vi "Process.vi"(8 "error in":errorcluster, 11 "Example Instrument UI":refnum<class "Instrument.PPMS UI.lvclass">) -> (0 "error out":errorcluster, 3 "Example Instrument UI out":refnum<class "Instrument.PPMS UI.lvclass">)   [LabVIEW 2016, in "Instrument.PPMS UI.lvclass"]
doc: "---------------------------------------------------------------\nJKI State Machine Objects™\nhttp://jki.net/state-machine-objects/\nCopyright (C) 2005-2015, JKI <info@jki.net>\nALL RIGHTS RESERVEDJKI State Machine Objects (SMO) 1.0.0.5\nJKI - JKI\nCopyright (c) 2016, JKI"
uses:
  Instrument.PPMS UI.lvclass
  C:/Program Files (x86)/National Instruments/LabVIEW 2016/vi.lib/JKI/JKI SMO/SMO/SMO.lvclass
  C:/Program Files (x86)/National Instruments/LabVIEW 2016/vi.lib/JKI/JKI SMO/SMO.UI/SMO.UI.lvclass
  instrument.PPMS/Typedefs/Magnet Status--PPMS--ring.ctl
  instrument.PPMS/Typedefs/Temperature Status--PPMS--ring.ctl
  <vilib>/JKI/JKI SMO/SMO/Typedefs/Parent Call--Enum.ctl
  instrument.PPMS/instrument.PPMS.lvclass
  C:/Program Files (x86)/National Instruments/LabVIEW 2016/user.lib/LevyLab/Levylab Instruments/SMOs/Instrument/Instrument.lvclass
  Instrument.PPMS UI.lvclass/Instrument.PPMS UI.ctl
  instrument.PPMS/Typedefs/getAll--PPMS--cluster.ctl
  <vilib>/JKI/JKI SMO/SMO.UI/SMO.UI.lvclass
  <vilib>/JKI/JKI SMO/SMO/SMO.lvclass
  <userlib>/LevyLab/Levylab Instruments/SMOs/Instrument/Instrument.lvclass
panel:
  in  "Field":bool
  in  "Temperature":bool
  in  "Target Field (Oe)":dbl=-0.00643419474363327 format="%_3g"
  in  "Target Temperature (K)":dbl=305.0156 format="%#_5g"
  out "PPMS 1 Temperature Status":T1 items=["TemperatureUnknown"=0, "Stable"=1, "Tracking"=2, "Near"=5, "Chasing"=6, "Filling"=7, "Standby"=10, "Disabled"=13, "ImpedanceNotFunction"=14, "TempFailure"=15]
  out "PPMS 1 Magnet Status":T2=1 items=["MagnetUnknown"=0, "StablePersistent"=1, "WarmingSwitch"=2, "CoolingSwitch"=3, "StableDriven"=4, "Iterating"=5, "Charging"=6, "Discharging"=7, "CurrentError"=8, "MagnetFailure"=15]
  out "Helium Level (%)":dbl=86.7
  out "Field (Oe)":dbl=-0.00643419474363327 format="%_3g"
  out "Temperature(K)":dbl=305.0156 format="%#_5g"
  in  "update time (ms)":u32=200
  in  "STOP":bool
  # "PPMS Monitor"
  # "SMO UI Template"
  # "For instructions on how to use the JKI State Machine Objects, examples and video tutorials, visit:\nhttp://jki.net/state-machine-objects/\n\nJKI State Machine Objects™\nhttp://jki.net/state-machine-objects/\nCopyright (C) 2005-2015, JKI <info@jki.net>\nALL RIGHTS RESERVED"
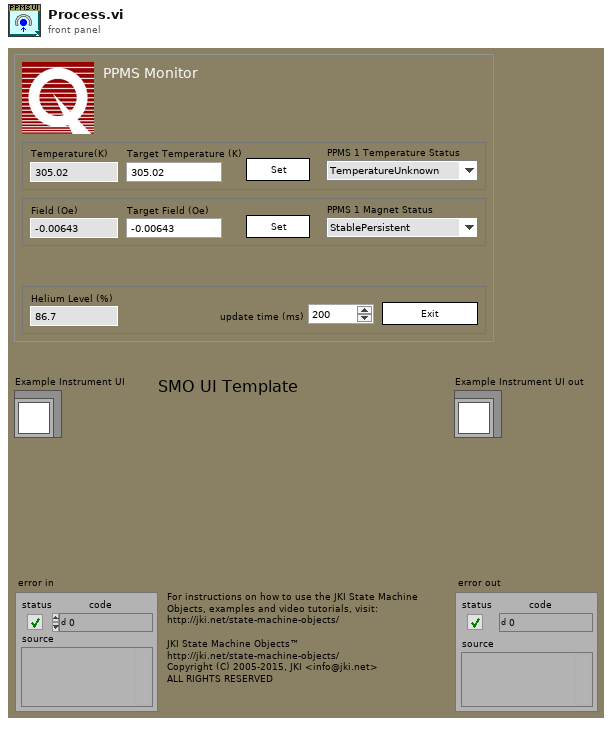
[diagram p1: front panel]
types:
  T1 = typedef "instrument.PPMS.lvclass/Temperature Status--PPMS--ring.ctl" = i32
  T2 = typedef "instrument.PPMS.lvclass/Magnet Status--PPMS--ring.ctl" = i32
  T3 = typedef "SMO.lvclass/Parent Call--Enum.ctl" = enum16{"Allows parent to run", "Does not request parent to run"}
  T4 = enum32{"invalid app kind", "Development System", "Run Time System", "Student Edition", "Embedded LabVIEW", "Evaluation", "Custom"}
  T5 = enum32{"Invalid", "Standard", "Closed", "Hidden", "Minimized", "Maximized"}
  T6 = typedef "instrument.PPMS.lvclass/getAll--PPMS--cluster.ctl" = cluster{"PPMS 1 Helium Level":dbl, "PPMS 1 Temperature":dbl, "PPMS 1 Temperature Status":T1, "PPMS 1 Magnetic Field":dbl, "PPMS 1 Magnet Status":T2}
  T7 = cluster{"Core":cluster{"Current VI Reference":refnum<vi>, "Close Panel on Exit?":bool, "error":errorcluster}, "Self Reference":refnum<class "Instrument.PPMS UI.lvclass">, "instrument.PPMS":refnum<class "instrument.PPMS.lvclass">, "Data Send":variant, "Data Receive":variant}
  T8 = cluster{"Current VI Reference":refnum<vi>, "Close Panel on Exit?":bool, "error":errorcluster}
  T9 = typedef "SMO.lvclass/Protected Events.ctl" = cluster{"StopProcesses":refnum<user-event>, "AbortProcesses":refnum<user-event>, "Config Changed":refnum<user-event>, "Dependency":refnum<user-event>}
  T10 = typedef "Instrument.lvclass/PublicEvents--Cluster.ctl" = cluster{"MessageFromProcess":refnum<user-event>}
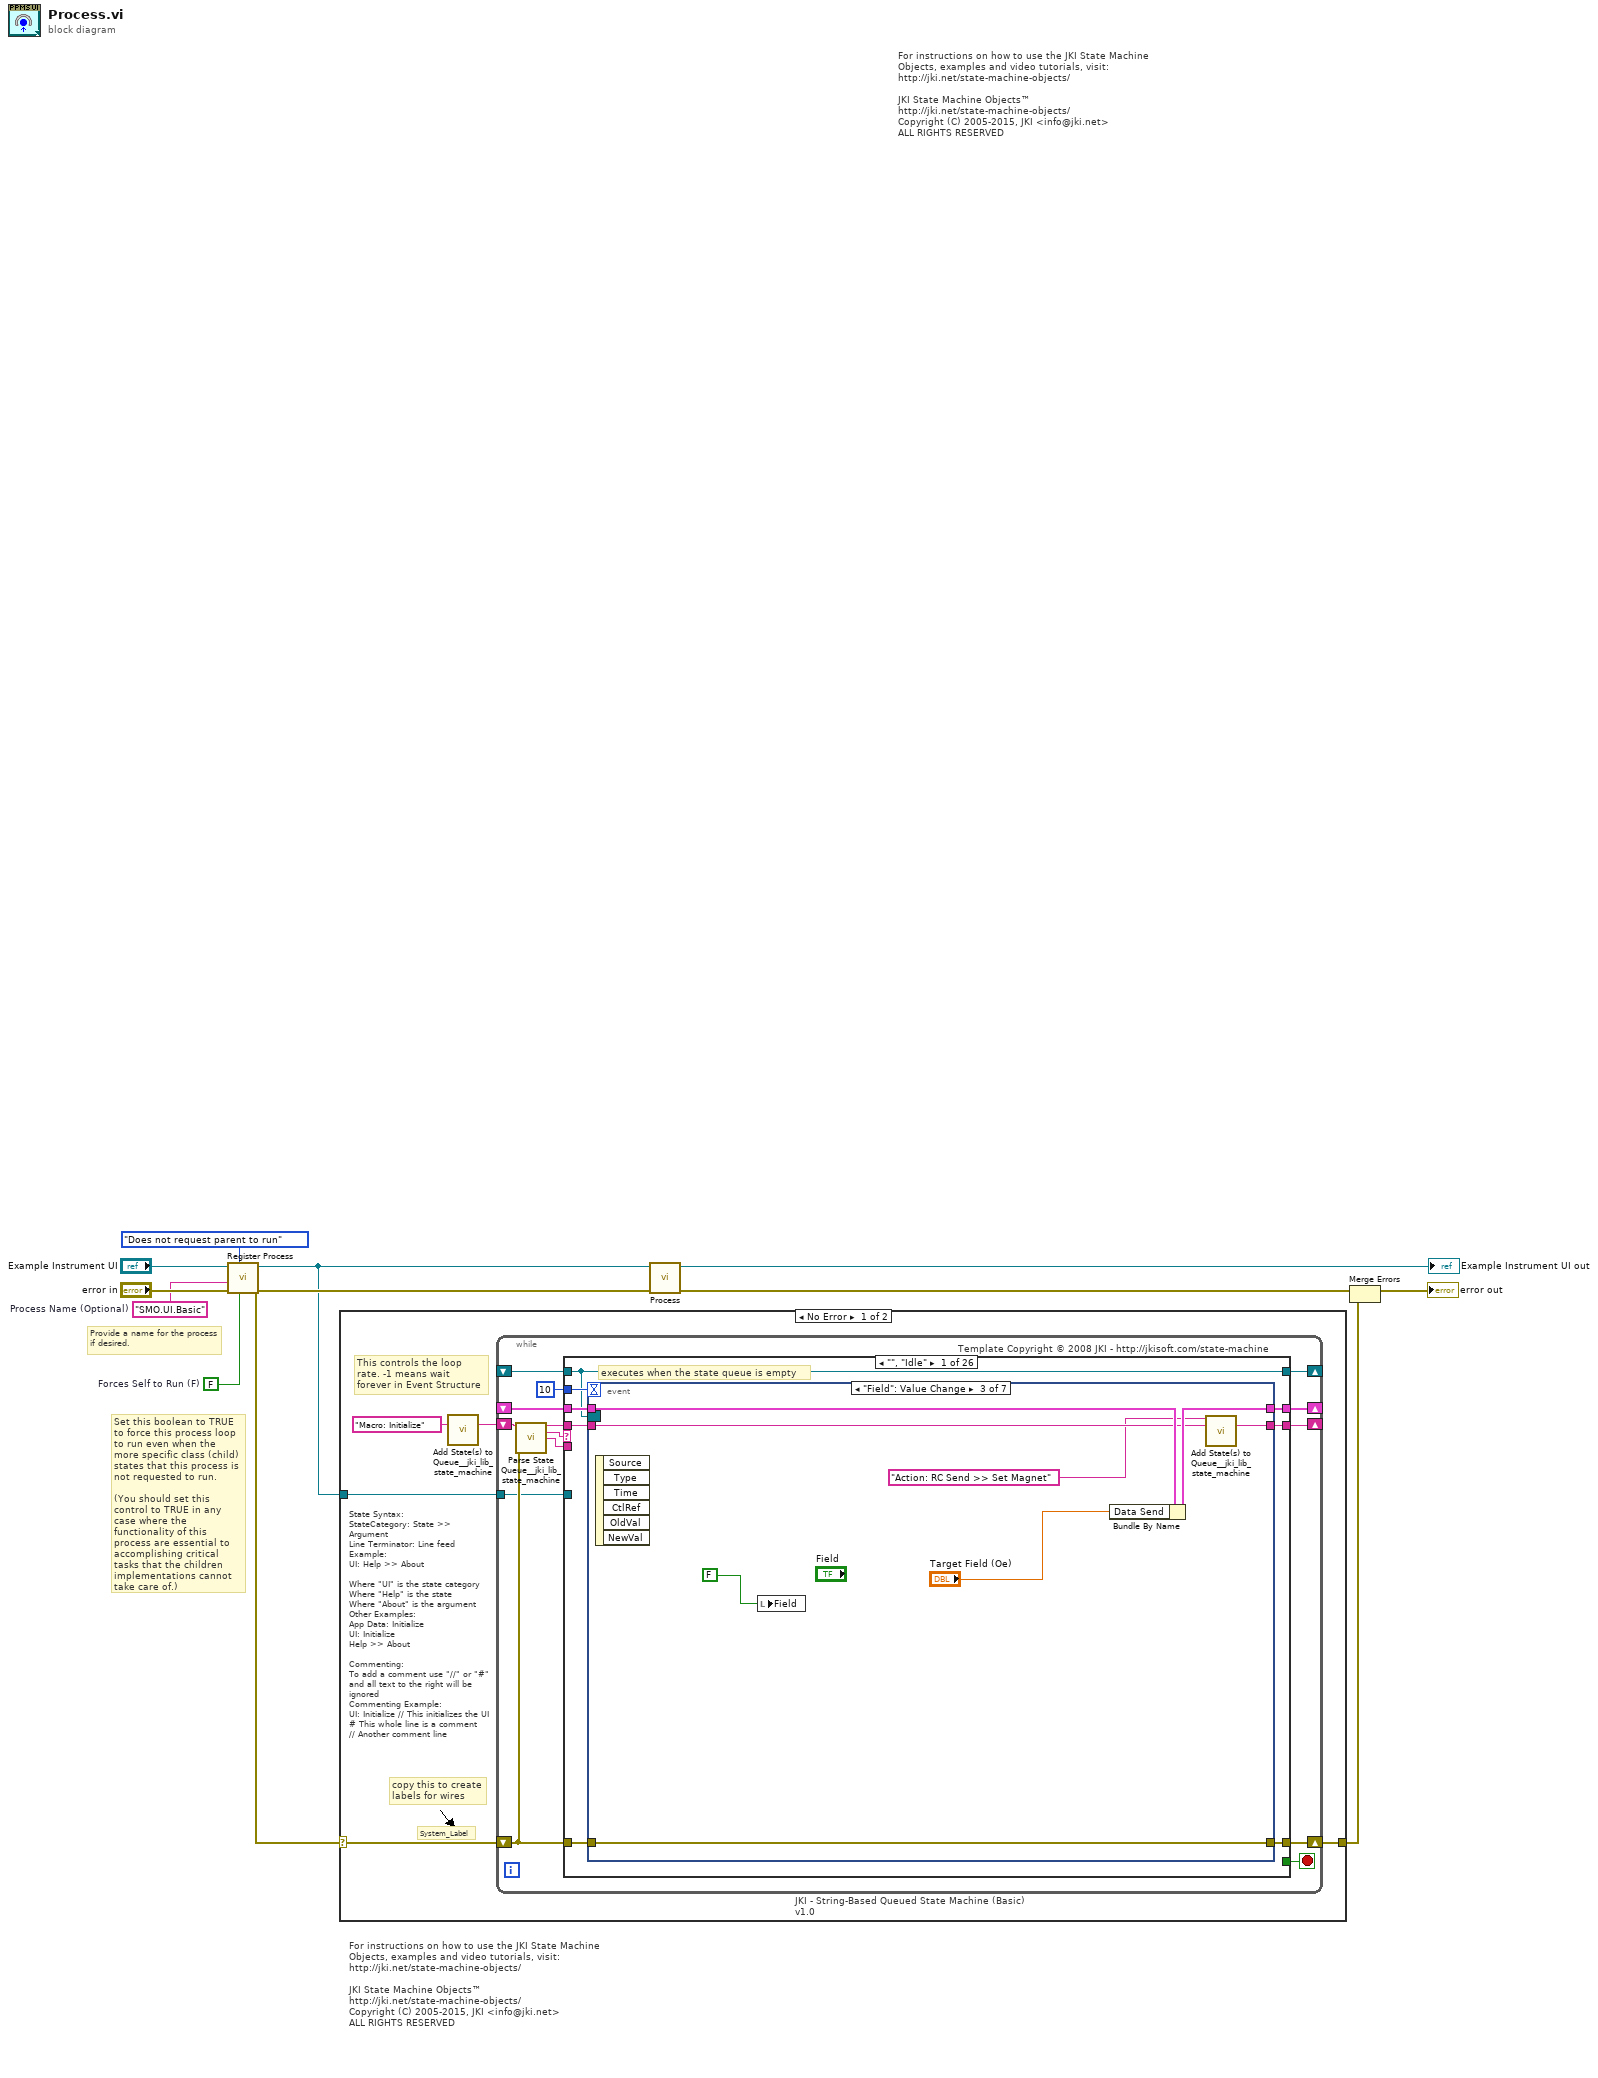
[diagram p0: block diagram]
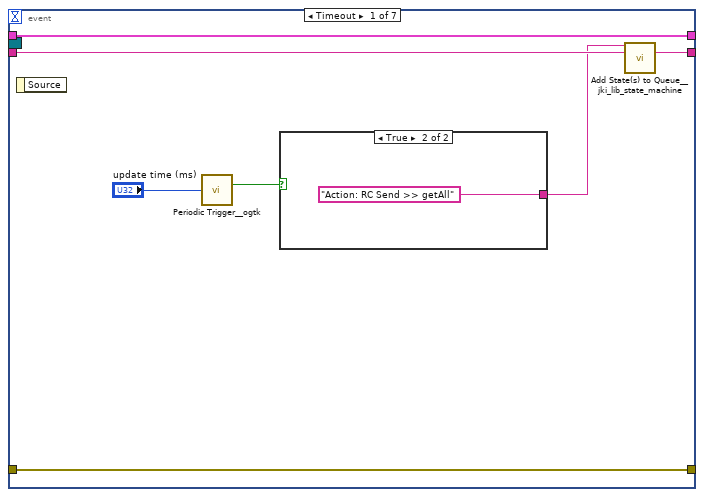
[diagram p2: hidden frame]
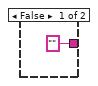
[diagram p3: hidden frame]
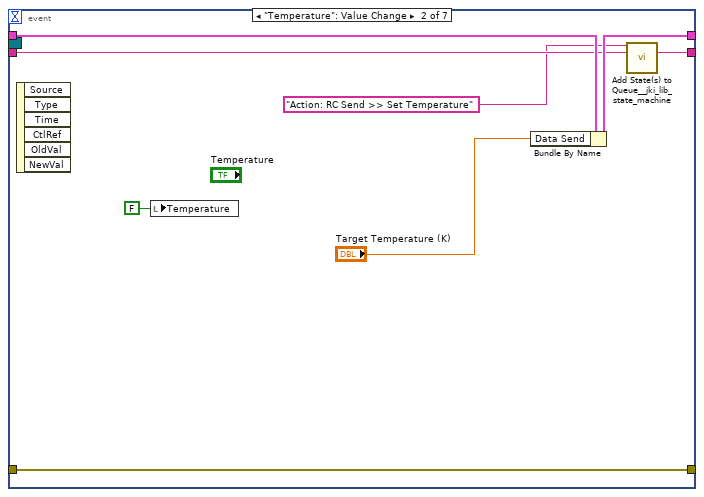
[diagram p4: hidden frame]
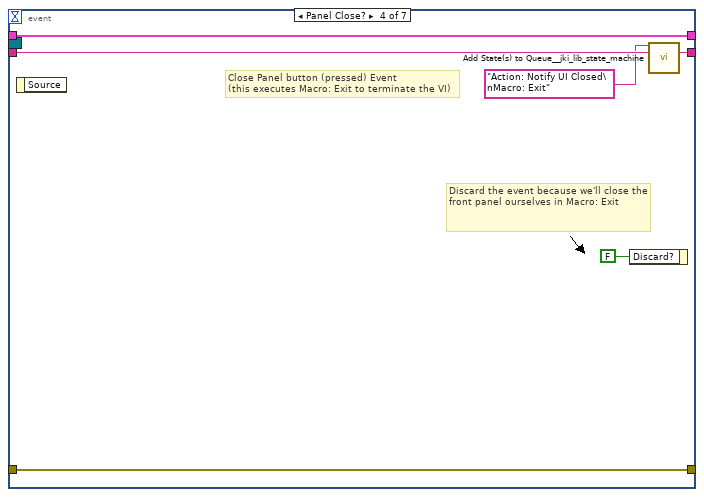
[diagram p5: hidden frame]
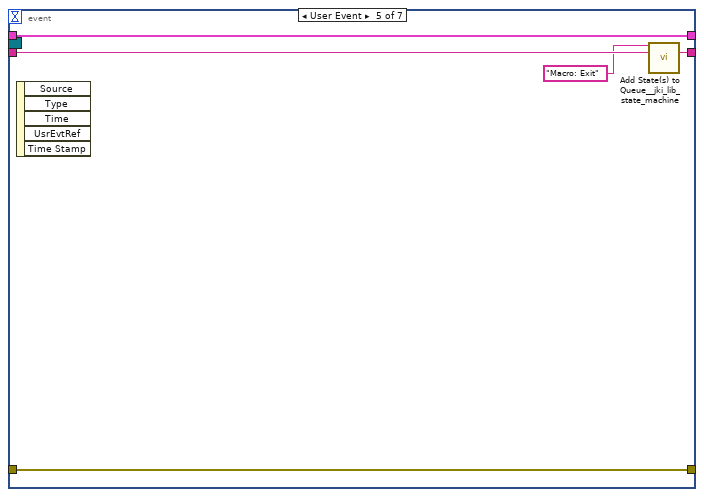
[diagram p6: hidden frame]
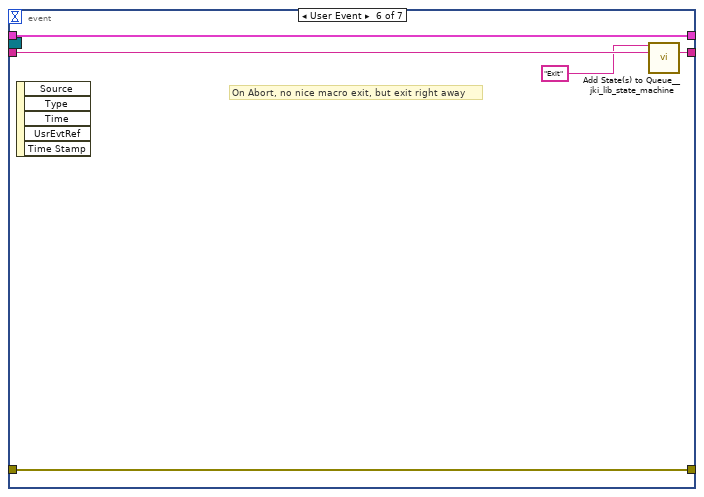
[diagram p7: hidden frame]
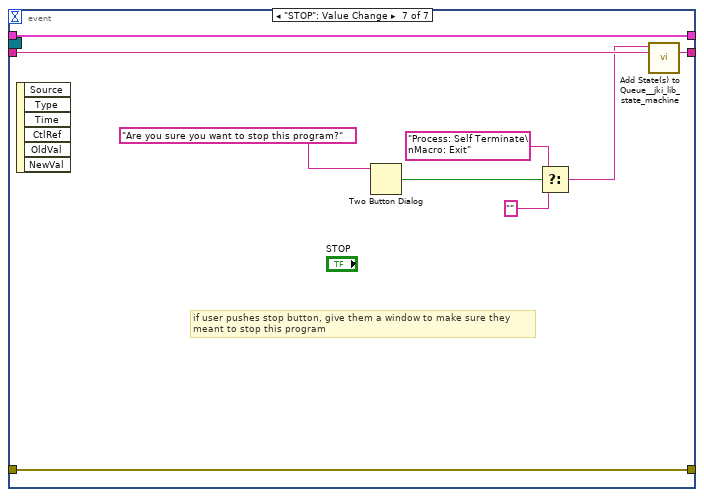
[diagram p8: hidden frame]
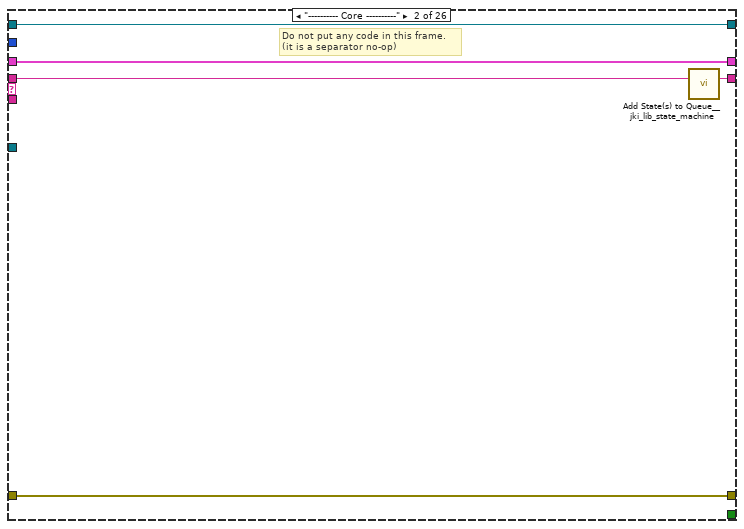
[diagram p9: hidden frame]
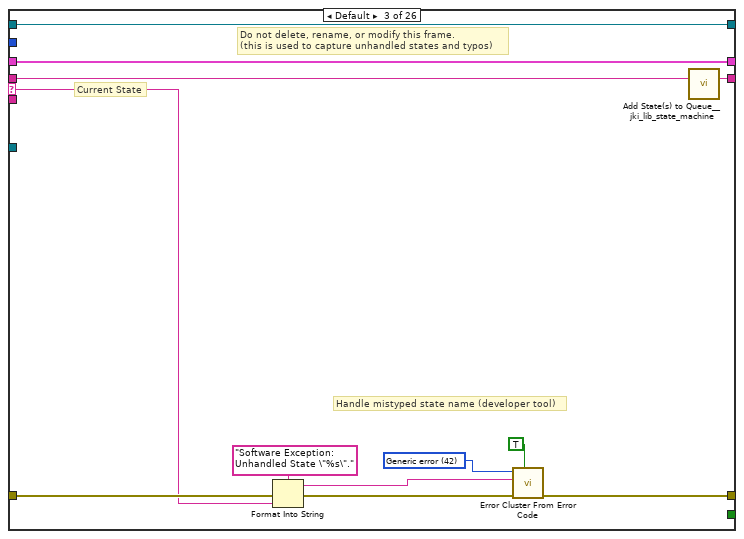
[diagram p10: hidden frame]
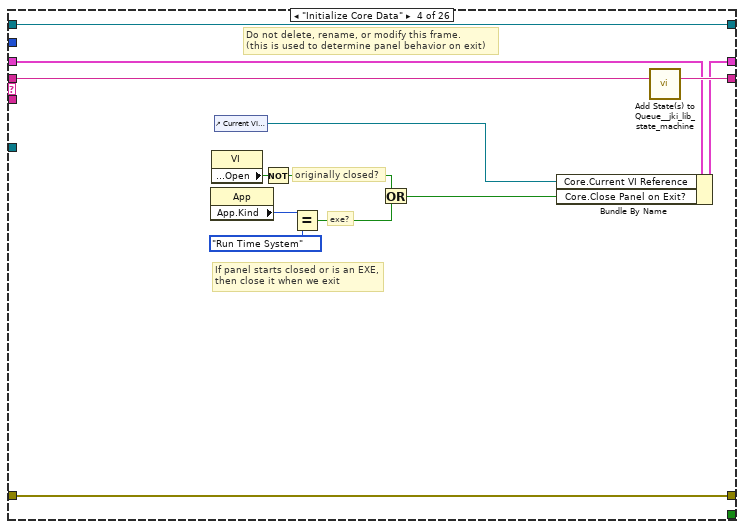
[diagram p11: hidden frame]
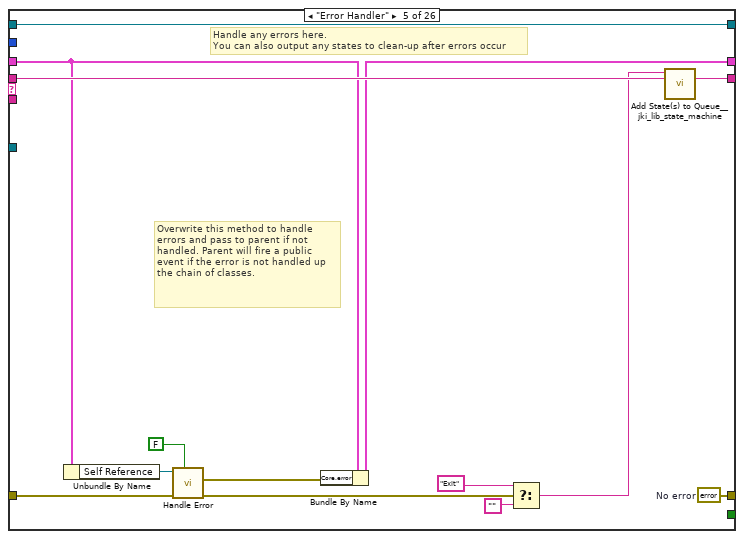
[diagram p12: hidden frame]
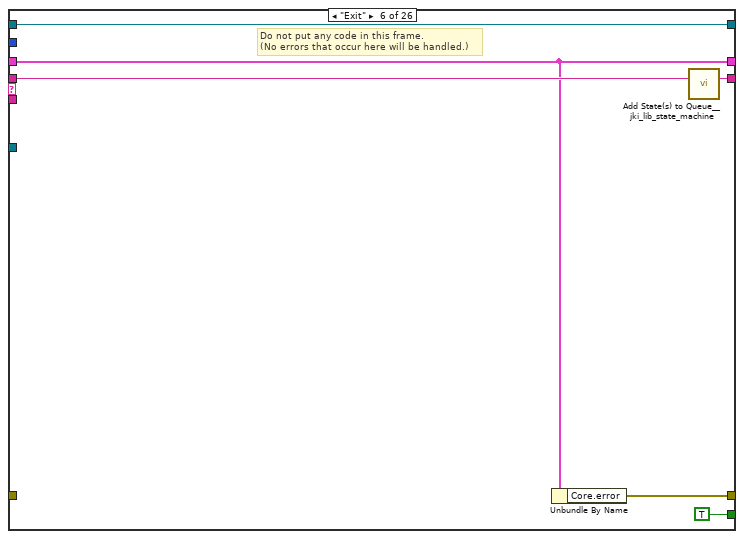
[diagram p13: hidden frame]
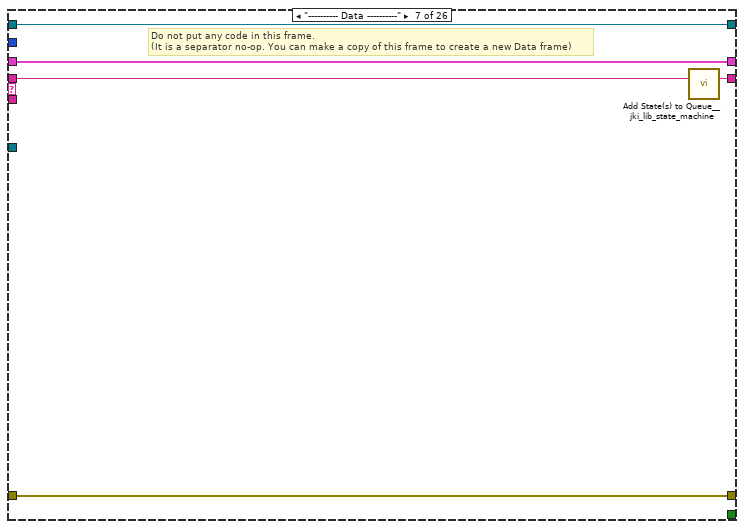
[diagram p14: hidden frame]
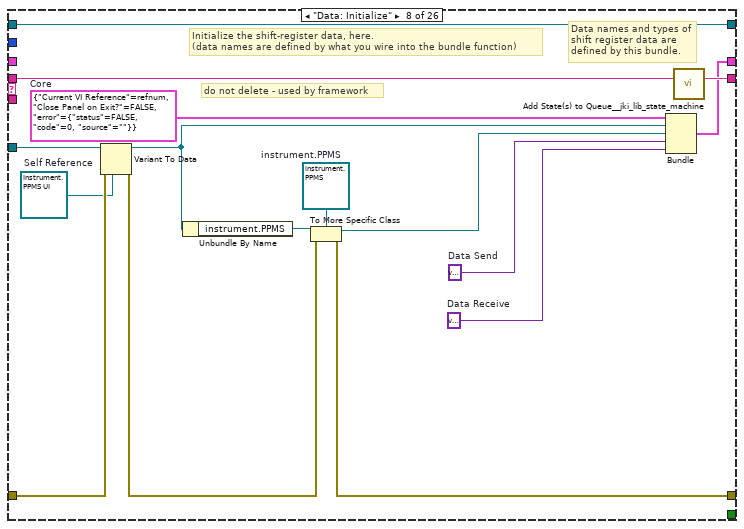
[diagram p15: hidden frame]
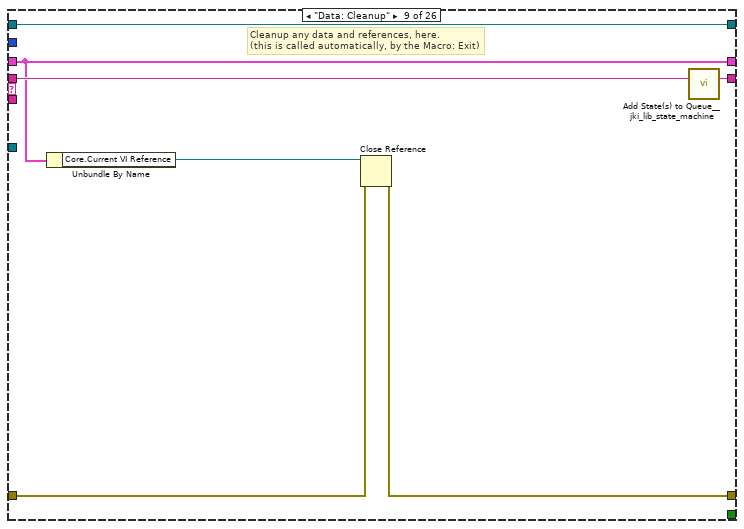
[diagram p16: hidden frame]
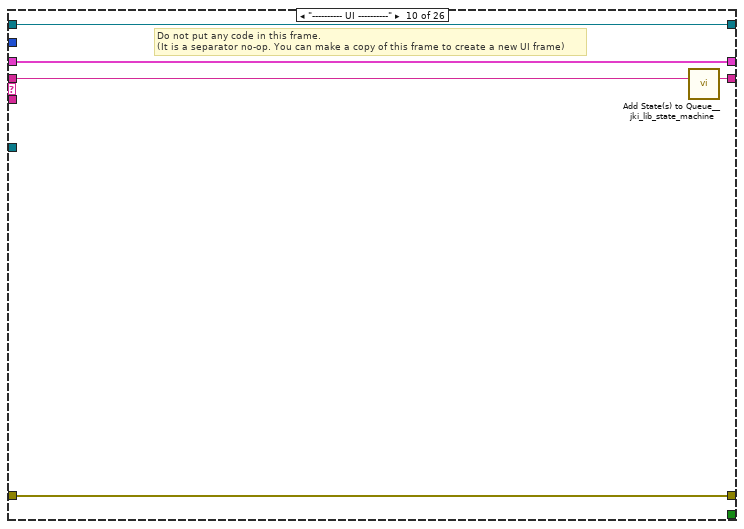
[diagram p17: hidden frame]
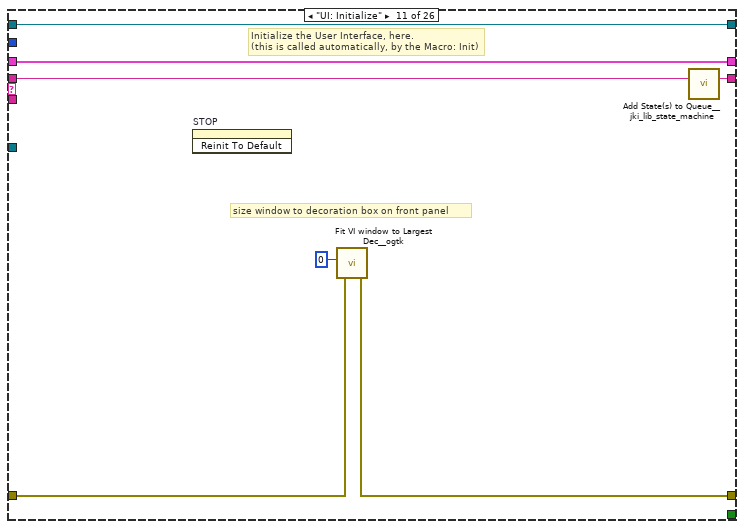
[diagram p18: hidden frame]
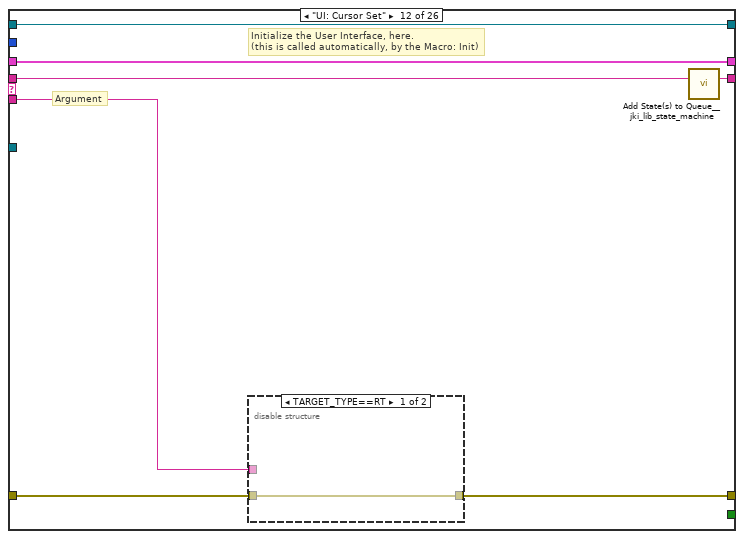
[diagram p19: hidden frame]
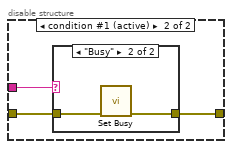
[diagram p20: hidden frame]
diagram:
  w2 = FALSE  # Forces Self to Run (F)
  w1 = "SMO.UI.Basic"  # Process Name (Optional)
  # "For instructions on how to use the JKI State Machine Objects, examples and video tutorials, visit:\nhttp://jki.net/state-machine-objects/\n\nJKI State Machine Objects™\nhttp://jki.net/state-machine-objects/\nCopyright (C) 2005-2015, JKI <info@jki.net>\nALL RIGHTS RESERVED"
  # "Provide a name for the process\nif desired."
  # "Set this boolean to TRUE to force this process loop to run even when the more specific class (child) states that this process is not requested to run.\n\n(You should set this control to TRUE in any case where the functionality of this process are essential to accomplishing critical tasks that the children implementations cannot take care of.)"
  # "For instructions on how to use the JKI State Machine Objects, examples and video tutorials, visit:\nhttp://jki.net/state-machine-objects/\n\nJKI State Machine Objects™\nhttp://jki.net/state-machine-objects/\nCopyright (C) 2005-2015, JKI <info@jki.net>\nALL RIGHTS RESERVED"
  n1 = call <vilib>:"Register Process.vi"("Forces Self to Run (F)"=w2, "Parent Call"=Parent_Call--Enum."Does not request parent to run", "error in (no error)"="error in", "Process Name (optional)"=w1, "SMO"="Example Instrument UI") -> ("error out"=w8:errorcluster, "SMO out"=w7:refnum<class "Instrument.PPMS UI.lvclass">)  [unwired: 5 in]
  n2 = case shown="No Error" w8 {
    selector: w8 -> [w13 w350]
    tunnel: w7 -> [w14 _]
    tunnel: [w12 w350] -> w4
    frame No Error {
      # "State Syntax:\nStateCategory: State >> Argument\nLine Terminator: Line feed\nExample:\nUI: Help >> About\n\nWhere \"UI\" is the state category\nWhere \"Help\" is the state\nWhere \"About\" is the argument\nOther Examples:\nApp Data: Initialize\nUI: Initialize\nHelp >> About\n\nCommenting:\nTo add a comment use \"//\" or \"#\" and all text to the right will be ignored\nCommenting Example:\nUI: Initialize // This initializes the UI\n# This whole line is a comment\n// Another comment line"
      # "copy this to create labels for wires"
      # "This controls the loop rate. -1 means wait forever in Event Structure"
      # "System_Label"
      n3 = call <vilib>:"Add State(s) to Queue__jki_lib_state_machine.vi"("State(s) in (\"\")"="Macro: Initialize") -> ("States Out"=w16:string)  [unwired: 14 in]
      n4 = while "JKI - String-Based Queued State Machine (Basic) v1.0" {
        shift-right: [w23] -> _
        shift-left: _ -> [w22]
        shift-right: [w26] -> w12
        shift-left: w13 -> [w20]
        shift-right: [w25] -> _
        shift-left: w16 -> [w27]
        tunnel: w14 -> [w19]
        shift-right: [w18] -> _
        shift-left: _ -> [w17]
        stop <- w24 stop-if-true
        # "Template Copyright © 2008 JKI - http://jkisoft.com/state-machine"
        n5 = call <vilib>:"Parse State Queue__jki_lib_state_machine.vi"("State Queue"=w27, "Error In (no error)"=w20) -> ("Remaining States"=w29:string, "Current State"=w30:string, "Arguments"=w28:string)  [unwired: 11 in]
        n6 = case shown="\"\", \"Idle\"" w30 {
          selector: w30 -> [_ _ w95 _ _ _ _ _ _ _ _ _ _ _ _ _ _ _ _ _ _ _ _ _ _ _]
          tunnel: w29 -> [w38 w93 w99 w118 w132 w138 w143 w159 w166 w171 w178 w185 w201 w233 w242 w256 w261 w272 w279 w284 w297 w303 w310 w317 w331 w345]
          tunnel: w28 -> [_ _ _ _ _ _ _ _ _ _ _ w179 w195 _ _ _ _ _ _ _ _ _ _ _ _ w336]
          tunnel: w22 -> [w36 w90 w97 w109 w120 w134 w140 _ w162 w168 w176 w183 w197 w230 w238 w247 w258 w269 w274 w281 w295 w301 w306 w313 w328 w342]
          tunnel: [w35 w91 w101 w115 w125 w133 w141 w145 w163 w169 w173 w180 w198 w231 w240 w254 w259 w263 w275 w282 w290 w298 w307 w311 w326 w334] -> w26
          tunnel: w20 -> [w34 w91 w100 w115 w121 _ w141 w156 w160 w169 w174 w181 w199 w231 w240 w254 w259 w264 w276 w282 w292 w299 w307 w312 w327 w335]
          tunnel: [w37 w92 w98 w117 w131 w137 w142 w158 w165 w170 w177 w184 w200 w232 w241 w255 w260 w271 w278 w283 w296 w302 w309 w316 w330 w344] -> w25
          tunnel: [_ _ _ _ _ TRUE _ _ _ _ _ _ _ _ _ _ _ _ _ _ _ _ _ _ _ _] -> w24
          tunnel: [w33 w90 w97 w116 w123 w134 w140 w157 w162 w168 w176 w183 w197 w230 w238 w247 w258 w269 w274 w281 w295 w301 w305 w313 w328 w341] -> w23
          tunnel: 10 ("Timeout") -> [w32 _ _ _ _ _ _ _ _ _ _ _ _ _ _ _ _ _ _ _ _ _ _ _ _ _]
          tunnel: w19 -> [_ _ _ _ _ _ _ w154 _ _ _ _ _ _ _ _ _ _ _ _ _ _ _ _ _ _]
          tunnel: [w31 w89 w94 w106 w130 w135 w139 w153 w161 w167 w175 w182 w194 w229 w239 w248 w257 w270 w277 w280 w294 w300 w308 w315 w329 w343] -> w18
          tunnel: w17 -> [w31 w89 w94 w106 w130 w135 w139 w153 w161 w167 w175 w182 w194 w229 w239 w248 w257 w270 w277 w280 _ w300 w308 w315 w329 w343]
          frame "", "Idle" {
            # "executes when the state queue is empty"
            n7 = event shown="[2] \"Field\": Value Change" {
              selector: w31 -> [_ _ _ _ _ _ _]
              dyn-events: _ -> [_ _ _ _ _ _ _]
              timeout: w32 -> [_ _ _ _ _ _ _]
              tunnel: w38 -> [w45 w51 w59 w69 w74 w79 w88]
              tunnel: [w44 w54 w62 w68 w73 w78 w87] -> w37
              tunnel: w36 -> [w42 w53 w61 w65 w71 w76 w85]
              tunnel: [w43 w55 w63 w64 w72 w77 w86] -> w35
              tunnel: w34 -> [w43 w55 w63 w64 w72 w77 w86]
              tunnel: [w42 w52 w60 w65 w71 w76 w85] -> w33
              event Timeout {
                n8 = event-data() -> ()  [unwired: 1 in, 1 out]
                n9 = call <userlib>:"Periodic Trigger__ogtk.vi"("time (ms)"="update time (ms)") -> ("Triggered"=w41:bool)  [unwired: 12 in, 2 out]
                n10 = case shown="True" w41 {
                  tunnel: ["" "Action: RC Send >> getAll"] -> w39
                  frame False {
                  }
                  frame True {
                  }
                }
                n11 = call <vilib>:"Add State(s) to Queue__jki_lib_state_machine.vi"("State(s) in Front (\"\")"=w39, "State(s) in (\"\")"=w45) -> ("States Out"=w44:string)  [unwired: 13 in]
              }
              event "Temperature": Value Change {
                n12 = event-data() -> ()  [unwired: 1 in, 6 out]
                n13 = local write "Temperature"(FALSE ("Temperature")) -> ()
                n14 = Bundle By Name(cluster=w53, "Data Send"="Target Temperature (K)") -> (w52:T7)
                n15 = call <vilib>:"Add State(s) to Queue__jki_lib_state_machine.vi"("State(s) in Front (\"\")"="Action: RC Send >> Set Temperature" ("State(s) in Front (\"\")"), "State(s) in (\"\")"=w51) -> ("States Out"=w54:string)  [unwired: 13 in]
              }
              event "Field": Value Change {
                n16 = event-data() -> ()  [unwired: 1 in, 6 out]
                n17 = local write "Field"(FALSE ("Field")) -> ()
                n18 = Bundle By Name(cluster=w61, "Data Send"="Target Field (Oe)") -> (w60:T7)
                n19 = call <vilib>:"Add State(s) to Queue__jki_lib_state_machine.vi"("State(s) in Front (\"\")"="Action: RC Send >> Set Magnet" ("State(s) in Front (\"\")"), "State(s) in (\"\")"=w59) -> ("States Out"=w62:string)  [unwired: 13 in]
              }
              event Panel Close? {
                # "Discard the event because we'll close the front panel ourselves in Macro: Exit"
                # "Close Panel button (pressed) Event\n(this executes Macro: Exit to terminate the VI)"
                n20 = event-data() -> ()  [unwired: 1 in, 1 out]
                n21 = event-data("Discard?"=FALSE) -> ()  [unwired: 1 in, 1 out]
                n22 = call <vilib>:"Add State(s) to Queue__jki_lib_state_machine.vi"("State(s) in Front (\"\")"="Action: Notify UI Closed\nMacro: Exit", "State(s) in (\"\")"=w69) -> ("States Out"=w68:string)  [unwired: 13 in]
              }
              event User Event {
                n23 = event-data() -> ()  [unwired: 1 in, 5 out]
                n24 = call <vilib>:"Add State(s) to Queue__jki_lib_state_machine.vi"("State(s) in Front (\"\")"="Macro: Exit", "State(s) in (\"\")"=w74) -> ("States Out"=w73:string)  [unwired: 13 in]
              }
              event User Event {
                # "On Abort, no nice macro exit, but exit right away"
                n25 = event-data() -> ()  [unwired: 1 in, 5 out]
                n26 = call <vilib>:"Add State(s) to Queue__jki_lib_state_machine.vi"("State(s) in Front (\"\")"="Exit", "State(s) in (\"\")"=w79) -> ("States Out"=w78:string)  [unwired: 13 in]
              }
              event "STOP": Value Change {
                # "if user pushes stop button, give them a window to make sure they\nmeant to stop this program"
                n27 = event-data() -> ()  [unwired: 1 in, 6 out]
                n28 = Two Button Dialog(message="Are you sure you want to stop this program?") -> (T button?=w84:bool)  [unwired: 2 in]
                n29 = Select(t="Process: Self Terminate\nMacro: Exit", s=w84, f="") -> (s? t:f=w80:string)
                n30 = call <vilib>:"Add State(s) to Queue__jki_lib_state_machine.vi"("State(s) in Front (\"\")"=w80, "State(s) in (\"\")"=w88) -> ("States Out"=w87:string)  [unwired: 13 in]
              }
            }
          }
          frame "---------- Core ----------" {
            # "Do not put any code in this frame.\n(it is a separator no-op)"
            n31 = call <vilib>:"Add State(s) to Queue__jki_lib_state_machine.vi"("State(s) in (\"\")"=w93) -> ("States Out"=w92:string)  [unwired: 14 in]
          }
          frame Default {
            w104 = 42 items=["No error", "Argument error", "Memory is full", "Out of zone", "End of file", "File already open", "Generic file I/O error", "File not found", "File permission error", "Disk is full", "Duplicate path", "Too many files open", "System feature not enabled", "Resource file not found", "Cannot add resource", "Resource not found", "Image not found", "Image memory error", "Pen does not exist", "Config type invalid", "Config token not found", "Config parse error", "Config memory error", "Bad external code format", "Bad external code offset", "External code not present", "Null window", "Destroy window error", "Null menu", "Print aborted", "Bad print record", "Print driver error", "Windows error during printing", "Memory error during printing", "Print dialog error", "Generic print error", "Invalid device refnum", "Device not found", "Device parameter error", "Device unit error", "Cannot open device", "Device call aborted", "Generic error", "Cancelled by user", "Object ID too low", "Object ID too high", "Object not in heap", "Unknown heap", "Unknown object (invalid DefProc)", "Unknown object (DefProc not in table)", "Message out of range", "Invalid (null) method", "Unknown message", "Manager call not supported", "Bad address", "Network operation in progress", "Network operation timed out", "Connection is busy", "Network attribute not supported", "Network error", "Address in use", "System out of memory", "Connection aborted", "Connection refused", "Not connected", "Already connected", "Connection closed", "Initialization error (interapplication manager)", "Bad occurrence", "Wait on unbound occurrence handler", "Occurrence queue overflow", "Datalog type conflict", "Unused", "Unrecognized type (interapplication manager)", "Memory corrupt", "Failed to make temporary DLL", "Old CIN version", "Drag socket not found", "Failed to load drop-object", "Failed to register OLE object", "Failed to release OLE object", "Format specifier type mismatch", "Unknown format specifier", "Too few format specifiers", "Too many format specifiers", "Scan failed", "Newer CIN version", "Error converting to variant", "Runtime menu error", "Password tampered", "Variant attribute not found", "Incompatible variant data type", "Event data is not available", "Event Store is not present", "Occurrence is not found", "Event Queue is not created", "Event info is not available", "Refnum passed is NULL", "Error retrieving Class GUID", "Error retrieving CoClass GUID", "Error retrieving TypeLib GUID.", "Bad built application magic bytes.", "Specific driver is different from the specific driver associated with the Logical Name.", "There is no session opened to the class driver.", "Max Error", "MAX - Error with config objects", "MAX - Error loading configuration", "MAX - Group not supported"]
            # "Current State"
            # "Do not delete, rename, or modify this frame.\n(this is used to capture unhandled states and typos)"
            # "Handle mistyped state name (developer tool)"
            n32 = Format Into String(format string="Software Exception: Unhandled State \"%s\"." ("message"), error in=w100, w95) -> (resulting string=w103:string, error out=w102:errorcluster)  [unwired: 1 in]
            n33 = call <vilib>:"Error Cluster From Error Code.vi"("show call chain? (False)"=TRUE, "error in (no error)"=w102, "error message (\"\")"=w103, "error code (0)"=w104) -> ("error out"=w101:errorcluster)  [unwired: 5 in]
            n34 = call <vilib>:"Add State(s) to Queue__jki_lib_state_machine.vi"("State(s) in (\"\")"=w99) -> ("States Out"=w98:string)  [unwired: 14 in]
          }
          frame "Initialize Core Data" {
            # "Do not delete, rename, or modify this frame.\n(this is used to determine panel behavior on exit)"
            # "originally closed?"
            # "exe?"
            # "If panel starts closed or is an EXE, then close it when we exit"
            n35 = property class="App"() -> ("App.Kind"=w113:T4)  [unwired: 2 in, 2 out]
            n36 = property class="VI"() -> ("Front Panel.Open"=w114:bool)  [unwired: 2 in, 2 out]
            n37 = control-ref of="Current VI Reference"() -> (w107:refnum<vi>)
            n38 = Not(x=w114) -> (.not. x?=w111:bool)
            n39 = Equal?(x=w113, y=T4."Run Time System" ("Application:Kind")) -> (x = y?=w110:bool)
            n40 = Or(x=w111, y=w110) -> (x .or. y?=w108:bool)
            n41 = Bundle By Name(cluster=w109, "Core.Current VI Reference"=w107, "Core.Close Panel on Exit?"=w108) -> (w116:T7)
            n42 = call <vilib>:"Add State(s) to Queue__jki_lib_state_machine.vi"("State(s) in (\"\")"=w118) -> ("States Out"=w117:string)  [unwired: 14 in]
          }
          frame "Error Handler" {
            w125 = errorcluster {"status"=FALSE, "code"=0, "source"=""}  # No error
            # "Overwrite this method to handle errors and pass to parent if not handled. Parent will fire a public event if the error is not handled up the chain of classes."
            # "Handle any errors here.\nYou can also output any states to clean-up after errors occur"
            n43 = Unbundle By Name(w120) -> ("Self Reference"=w129:refnum<class "Instrument.PPMS UI.lvclass">)
            n44 = call-dynamic "Handle Error.vi"("Stop on Unhandled Error (T)"=FALSE, "error in"=w121, "SMO"=w129) -> ("handling error"=w119:errorcluster, "Unhandled error"=w124:errorcluster)  [unwired: 6 in, 1 out]
            n45 = Bundle By Name(cluster=w120, "Core.error"=w124) -> (w123:T7)
            n46 = Select(t="Exit", s=w119, f="") -> (s? t:f=w126:string)
            n47 = call <vilib>:"Add State(s) to Queue__jki_lib_state_machine.vi"("State(s) in Front (\"\")"=w126, "State(s) in (\"\")"=w132) -> ("States Out"=w131:string)  [unwired: 13 in]
          }
          frame "Exit" {
            # "Do not put any code in this frame.\n(No errors that occur here will be handled.)"
            n48 = Unbundle By Name(w134) -> ("Core.error"=w133:errorcluster)
            n49 = call <vilib>:"Add State(s) to Queue__jki_lib_state_machine.vi"("State(s) in (\"\")"=w138) -> ("States Out"=w137:string)  [unwired: 14 in]
          }
          frame "---------- Data ----------" {
            # "Do not put any code in this frame.\n(It is a separator no-op. You can make a copy of this frame to create a new Data frame)"
            n50 = call <vilib>:"Add State(s) to Queue__jki_lib_state_machine.vi"("State(s) in (\"\")"=w143) -> ("States Out"=w142:string)  [unwired: 14 in]
          }
          frame "Data: Initialize" {
            w144 = variant  # Data Receive
            w149 = refnum<class "instrument.PPMS.lvclass"> refnum  # instrument.PPMS
            w150 = variant  # Data Send
            w152 = T8 {"Current VI Reference"=refnum, "Close Panel on Exit?"=FALSE, "error"={"status"=FALSE, "code"=0, "source"=""}}  # Core
            w155 = refnum<class "Instrument.PPMS UI.lvclass"> refnum  # Self Reference
            # "do not delete - used by framework"
            # "Data names and types of shift register data are defined by this bundle."
            # "Initialize the shift-register data, here.\n(data names are defined by what you wire into the bundle function)"
            n51 = Variant To Data(error in=w156, type=w155, Variant=w154) -> (data=w151:refnum<class "Instrument.PPMS UI.lvclass">, error out=w146:errorcluster)
            n52 = Unbundle By Name(w151) -> ("instrument.PPMS"=w148:refnum<class "instrument.PPMS.lvclass">)
            n53 = To More Specific Class(target class=w149, reference=w148, error in=w146) -> (specific class reference=w147:refnum<class "instrument.PPMS.lvclass">, error out=w145:errorcluster)
            n54 = Bundle("Core"=w152, "Self Reference"=w151, "instrument.PPMS"=w147, "Data Send"=w150, "Data Receive"=w144) -> (w157:T7)  [unwired: 1 in]
            n55 = call <vilib>:"Add State(s) to Queue__jki_lib_state_machine.vi"("State(s) in (\"\")"=w159) -> ("States Out"=w158:string)  [unwired: 14 in]
          }
          frame "Data: Cleanup" {
            # "Cleanup any data and references, here.\n(this is called automatically, by the Macro: Exit)"
            n56 = Unbundle By Name(w162) -> ("Core.Current VI Reference"=w164:refnum<vi>)
            n57 = Close Reference(reference=w164, error in (no error)=w160) -> (error out=w163:errorcluster)
            n58 = call <vilib>:"Add State(s) to Queue__jki_lib_state_machine.vi"("State(s) in (\"\")"=w166) -> ("States Out"=w165:string)  [unwired: 14 in]
          }
          frame "---------- UI ----------" {
            # "Do not put any code in this frame.\n(It is a separator no-op. You can make a copy of this frame to create a new UI frame)"
            n59 = call <vilib>:"Add State(s) to Queue__jki_lib_state_machine.vi"("State(s) in (\"\")"=w171) -> ("States Out"=w170:string)  [unwired: 14 in]
          }
          frame "UI: Initialize" {
            # "size window to decoration box on front panel"
            # "Initialize the User Interface, here.\n(this is called automatically, by the Macro: Init)"
            n60 = invoke on="STOP" class="Bool (strict)" method="Reinit To Default"() -> ()  [unwired: 3 in, 3 out]
            n61 = call <userlib>:"Fit VI window to Largest Dec__ogtk.vi"("error in (no error)"=w174, "border spacing (2 px)"=0) -> ("error out"=w173:errorcluster)  [unwired: 4 in, 1 out]
            n62 = call <vilib>:"Add State(s) to Queue__jki_lib_state_machine.vi"("State(s) in (\"\")"=w178) -> ("States Out"=w177:string)  [unwired: 14 in]
          }
          frame "UI: Cursor Set" {
            # "Argument"
            # "Initialize the User Interface, here.\n(this is called automatically, by the Macro: Init)"
            n63 = disable-structure shown="TARGET_TYPE==RT" {
              disable-tunnel: w181 -> [w186 w189]
              disable-tunnel: [w186 w188] -> w180
              disable-tunnel: w179 -> [_ w187]
              frame condition #0 {
              }
              frame condition #1 (active) {
                n64 = case shown="\"Busy\"" w187 {
                  tunnel: w189 -> [w191 w193]
                  tunnel: [w190 w192] -> w188
                  frame "Idle", Default {
                    n65 = call <vilib>:"Unset Busy.vi"("error in (no error)"=w191) -> ("error out"=w190:errorcluster)  [unwired: 10 in]
                  }
                  frame "Busy" {
                    n66 = call <vilib>:"Set Busy.vi"("error in (no error)"=w193) -> ("error out"=w192:errorcluster)  [unwired: 9 in, 1 out]
                  }
                }
              }
            }
            n67 = call <vilib>:"Add State(s) to Queue__jki_lib_state_machine.vi"("State(s) in (\"\")"=w185) -> ("States Out"=w184:string)  [unwired: 14 in]
          }
          frame "UI: Front Panel State" {
            # "Argument"
            # "Set Front Panel Open or Closed\n(Usage: \"UI: Front Panel State >> Open|Close\")"
            n68 = Unbundle By Name(w197) -> ("Core.Current VI Reference"=w196:refnum<vi>)
            n69 = disable-structure shown="Default" {
              disable-tunnel: w199 -> [w205 w228]
              disable-tunnel: [w204 w228] -> w198
              disable-tunnel: w196 -> [w203 _]
              disable-tunnel: w195 -> [w202 _]
              frame condition #0 (active) {
                n70 = case shown="\"Close\"" w202 {
                  tunnel: w205 -> [w209 w222]
                  tunnel: [w211 w223] -> w204
                  tunnel: w203 -> [w210 w220]
                  frame "Open", Default {
                    n71 = property class="VI"(reference=w210, error in=w209) -> (reference out=w207:refnum<vi>, error out=w208:errorcluster, "FP.State"=w206:T5)
                    n72 = case shown="\"Closed\"" w206 {
                      tunnel: [w214 w217] -> w211
                      tunnel: w208 -> [w213 w217]
                      tunnel: w207 -> [w212 _]
                      frame "Closed" {
                        n73 = invoke class="VI" method="FP.Open"(reference=w212, error in=w213, "Activate"=TRUE, "State"=T5."Standard") -> (error out=w214:errorcluster)  [unwired: 1 in, 4 out]
                      }
                      frame Default {
                      }
                    }
                  }
                  frame "Close" {
                    n74 = property class="VI"(reference=w220, error in=w222) -> (reference out=w219:refnum<vi>, error out=w221:errorcluster, "FP.State"=w218:T5)
                    n75 = case shown="Default" w218 {
                      tunnel: [w224 w227] -> w223
                      tunnel: w221 -> [w224 w226]
                      tunnel: w219 -> [_ w225]
                      frame "Invalid", "Closed" {
                      }
                      frame Default {
                        n76 = invoke class="VI" method="FP.Close"(reference=w225, error in=w226) -> (error out=w227:errorcluster)  [unwired: 1 in, 2 out]
                      }
                    }
                  }
                }
              }
              frame condition #1 {
              }
            }
            n77 = call <vilib>:"Add State(s) to Queue__jki_lib_state_machine.vi"("State(s) in (\"\")"=w201) -> ("States Out"=w200:string)  [unwired: 14 in]
          }
          frame "---------- Macro ----------" {
            # "Do not put any code in this frame.\n(It is a separator no-op. You can make a copy of this frame to create a new Macro frame)"
            n78 = call <vilib>:"Add State(s) to Queue__jki_lib_state_machine.vi"("State(s) in (\"\")"=w233) -> ("States Out"=w232:string)  [unwired: 14 in]
          }
          frame "Macro: Initialize" {
            # "Initialization Macro\n(This is called once, when the VI starts)"
            n79 = call <vilib>:"Add State(s) to Queue__jki_lib_state_machine.vi"("State(s) in Front (\"\")"="Data: Initialize\nInitialize Core Data\nEvents: Register", "State(s) in (\"\")"="Process: Sync", "State(s) at Back (\"\")"="UI: Initialize\nUI: Front Panel State >> Open") -> ("States Out"=w235:string)  [unwired: 12 in]
            n80 = call <vilib>:"Add State(s) to Queue__jki_lib_state_machine.vi"("State(s) in Front (\"\")"=w235, "State(s) in (\"\")"=w242) -> ("States Out"=w241:string)  [unwired: 13 in]
          }
          frame "Macro: Exit" {
            # "Exit Macro\n(This is called once, when the VI exits)"
            n81 = Unbundle By Name(w247) -> ("Core.Close Panel on Exit?"=w253:bool)
            n82 = Select(t="UI: Front Panel State >> Close", s=w253, f="") -> (s? t:f=w250:string)
            n83 = call <vilib>:"Add State(s) to Queue__jki_lib_state_machine.vi"("State(s) in Front (\"\")"="Data: Cleanup\nEvents: Unregister", "State(s) in (\"\")"="Process: Sync", "State(s) at Back (\"\")"="Exit") -> ("States Out"=w244:string)  [unwired: 12 in]
            n84 = call <vilib>:"Add State(s) to Queue__jki_lib_state_machine.vi"("State(s) in (\"\")"=w250, "State(s) at Back (\"\")"=w244) -> ("States Out"=w249:string)  [unwired: 13 in]
            n85 = call <vilib>:"Add State(s) to Queue__jki_lib_state_machine.vi"("State(s) in Front (\"\")"=w249, "State(s) in (\"\")"=w256) -> ("States Out"=w255:string)  [unwired: 13 in]
          }
          frame "---------- Process ----------" {
            # "Template Separator\n(You can make a copy of, or modify, this frame)"
            n86 = call <vilib>:"Add State(s) to Queue__jki_lib_state_machine.vi"("State(s) in (\"\")"=w261) -> ("States Out"=w260:string)  [unwired: 14 in]
          }
          frame "Process: Sync" {
            n87 = Unbundle By Name(w269) -> ("Self Reference"=w265:refnum<class "Instrument.PPMS UI.lvclass">)
            n88 = call <vilib>:"WaitOnProcessSync.vi"("error in (no error)"=w264, "SMO"=w265) -> ("error out"=w263:errorcluster, "Don't run?"=w268:bool)  [unwired: 7 in, 1 out]
            n89 = Select(t="Data: Cleanup\nEvents: Unregister\nExit", s=w268, f="") -> (s? t:f=w262:string)
            n90 = call <vilib>:"Add State(s) to Queue__jki_lib_state_machine.vi"("State(s) in Front (\"\")"=w262, "State(s) in (\"\")"=w272) -> ("States Out"=w271:string)  [unwired: 13 in]
          }
          frame "Process: Self Terminate" {
            n91 = Unbundle By Name(w274) -> ("Self Reference"=w273:refnum<class "Instrument.PPMS UI.lvclass">)
            n92 = call <vilib>:"SelfTerminate.vi"("error in (no error)"=w276, "SMO in"=w273) -> ("error out"=w275:errorcluster)  [unwired: 8 in, 1 out]
            n93 = call <vilib>:"Add State(s) to Queue__jki_lib_state_machine.vi"("State(s) in (\"\")"=w279) -> ("States Out"=w278:string)  [unwired: 14 in]
          }
          frame "---------- Events ----------" {
            # "Template Separator\n(You can make a copy of, or modify, this frame)"
            n94 = call <vilib>:"Add State(s) to Queue__jki_lib_state_machine.vi"("State(s) in (\"\")"=w284) -> ("States Out"=w283:string)  [unwired: 14 in]
          }
          frame "Events: Register" {
            # "Expand to add\nmore events"
            # "Base Class Protected Events"
            n95 = Unbundle By Name(w295) -> ("Self Reference"=w288:refnum<class "Instrument.PPMS UI.lvclass">, "instrument.PPMS"=w287:refnum<class "instrument.PPMS.lvclass">)
            n96 = call <vilib>:"GetProtectedEvents.vi"("SMO"=w288) -> ("error out"=w289:errorcluster, "SMO Protected Events"=w293:T9)  [unwired: 8 in, 1 out]
            n97 = call <userlib>:"Instrument.GetPublicEvents.vi"("Instrument"=w287) -> ("error out"=w285:errorcluster, "Instrument Public Events"=w286:T10)  [unwired: 8 in, 1 out]
            n98 = register-events(w293, w286) -> (reference out=w294:refnum<event-registration>, error out=w291:errorcluster)  [unwired: 2 in]
            n99 = Merge Errors(w285, w292, w291, w289) -> (w290:errorcluster)
            n100 = call <vilib>:"Add State(s) to Queue__jki_lib_state_machine.vi"("State(s) in (\"\")"=w297) -> ("States Out"=w296:string)  [unwired: 14 in]
          }
          frame "Events: Unregister" {
            n101 = Unregister For Events(event registration refnum=w300, error in=w299) -> (error out=w298:errorcluster)
            n102 = call <vilib>:"Add State(s) to Queue__jki_lib_state_machine.vi"("State(s) in (\"\")"=w303) -> ("States Out"=w302:string)  [unwired: 14 in]
          }
          frame "---------- Action ----------" {
            n103 = Unbundle By Name(w306) -> ("Self Reference"=w304:refnum<class "Instrument.PPMS UI.lvclass">)
            n104 = Bundle By Name(cluster=w306, "Self Reference"=w304) -> (w305:T7)
            n105 = call <vilib>:"Add State(s) to Queue__jki_lib_state_machine.vi"("State(s) in (\"\")"=w310) -> ("States Out"=w309:string)  [unwired: 14 in]
          }
          frame "Action: Notify UI Closed" {
            # "Notify that the UI has been closed"
            n106 = Unbundle By Name(w313) -> ("Self Reference"=w314:refnum<class "Instrument.PPMS UI.lvclass">)
            n107 = call <vilib>:"Hide.vi"("error in (no error)"=w312, "SMO.UI"=w314) -> ("error out"=w311:errorcluster)  [unwired: 8 in, 1 out]
            n108 = call <vilib>:"Add State(s) to Queue__jki_lib_state_machine.vi"("State(s) in (\"\")"=w317) -> ("States Out"=w316:string)  [unwired: 14 in]
          }
          frame "Action: Update Front Panel All" {
            n109 = Unbundle By Name(w328) -> ("Data Receive"=w325:variant)
            n110 = Variant To Data(error in=w327, type=T6 {"PPMS 1 Helium Level"=0.0, "PPMS 1 Temperature"=0.0, "PPMS 1 Temperature Status"=0, "PPMS 1 Magnetic Field"=0.0, "PPMS 1 Magnet Status"=1} ("getAll"), Variant=w325) -> (data=w323:T6, error out=w326:errorcluster)
            n111 = Unbundle By Name(w323) -> ("PPMS 1 Helium Level"=→"Helium Level (%)":dbl, "PPMS 1 Temperature"=→"Temperature(K)":dbl, "PPMS 1 Temperature Status"=→"PPMS 1 Temperature Status":T1, "PPMS 1 Magnetic Field"=→"Field (Oe)":dbl, "PPMS 1 Magnet Status"=→"PPMS 1 Magnet Status":T2)
            n112 = call <vilib>:"Add State(s) to Queue__jki_lib_state_machine.vi"("State(s) in (\"\")"=w331) -> ("States Out"=w330:string)  [unwired: 14 in]
          }
          frame "Action: RC Send" {
            n113 = Unbundle By Name(w342) -> ("instrument.PPMS"=w338:refnum<class "instrument.PPMS.lvclass">, "Data Send"=w337:variant)
            n114 = call "PPMS Client.vi"("error in (no error)"=w335, "Data"=w337, "Command"=w336, "instrument.PPMS2 in"=w338) -> ("error out"=w334:errorcluster, "Data out"=w333:variant, "Command out"=w332:string)  [unwired: 4 in, 1 out]
            n115 = case shown="\"getAll\"" w332 {
              tunnel: ["" "Action: Update Front Panel All"] -> w340
              tunnel: w333 -> [_ w348]
              tunnel: [variant ("Data") w348] -> w339
              frame Default {
              }
              frame "getAll" {
              }
            }
            n116 = Bundle By Name(cluster=w342, "Data Receive"=w339) -> (w341:T7)
            n117 = call <vilib>:"Add State(s) to Queue__jki_lib_state_machine.vi"("State(s) in Front (\"\")"=w340, "State(s) in (\"\")"=w345) -> ("States Out"=w344:string)  [unwired: 13 in]
          }
        }
      }
    }
    frame Error {
    }
  }
  n118 = call-parent "Process.vi"("error in (no error)"=w8, "SMO.UI"=w7) -> ("error out"=w5:errorcluster, "SMO.UI out"=→"Example Instrument UI out":refnum<class "Instrument.PPMS UI.lvclass">)  [unwired: 8 in]
  n119 = Merge Errors(w5, w4) -> (→"error out":errorcluster)
